vi "BUILD_uninstall.vi"() -> ()   [LabVIEW 2013]
panel:
  out "error out":errorcluster
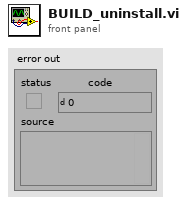
[diagram p1: front panel]
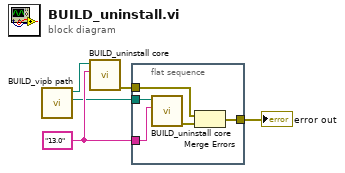
[diagram p0: block diagram]
diagram:
  w2 = "13.0" ("LabVIEW Version")
  n1 = call "BUILD_vipb path.vi"() -> ("2"=w1:path, "appended path"=w5:path)  [unwired: 10 in]
  n2 = call "BUILD_uninstall core.vi"("LabVIEW Version"=w2, "appended path"=w5) -> ("error out"=w4:errorcluster)  [unwired: 9 in]
  n3 = flat-sequence {
    tunnel: w4 -> [w10]
    tunnel: [w9] -> w3
    tunnel: w1 -> [w7]
    tunnel: w2 -> [w6]
    frame #0 {
      n4 = call "BUILD_uninstall core.vi"("LabVIEW Version"=w6, "appended path"=w7) -> ("error out"=w8:errorcluster)  [unwired: 9 in]
      n5 = Merge Errors(w10, w8) -> (w9:errorcluster)
    }
  }
  "error out" <- w3
